vi "Update_TL_Init_Values.vi"() -> ()   [LabVIEW 2012]
uses:
  <vilib>/Utility/config.llb/Read Key (Double).vi
  <vilib>/Utility/config.llb/Write Key (Double).vi
  <vilib>/Utility/config.llb/NI_LVConfig.lvlib
panel:
  in  "Update Button":bool
  out "TL Init Values":string[](array[string])
  out "Listed\nLog Entries":string
  out "FileSize":i64
  in  "Init File Path":path=path "C:/Users/eol-lidar/Desktop/ThorLabsLog Folder/h2o_dial_settings-2.txt"
  out "bytes/line":i64
  out "FilePosition":i64
  in  "Stop":bool
  in  "Next":bool
  in  "Previous":bool
  out "ThorLabs Log Entries":string[](array[string])
  in  "ETO(mS)":i32
  in  "TL Log Entry to Write into Init File":i32=5 min=1 max=5 step=1
  out "Total\nLog Entries":dbl
  out "Error Out":errorcluster
  in  "Error In":errorcluster
  in  "TL Log File":path=path "C:/Users/eol-lidar/Desktop/ThorLabsLog Folder/TL.log"
  # "Update ThorLab Init Values"
  # "1"
  # "2"
  # "3"
  # "4"
  # "5"
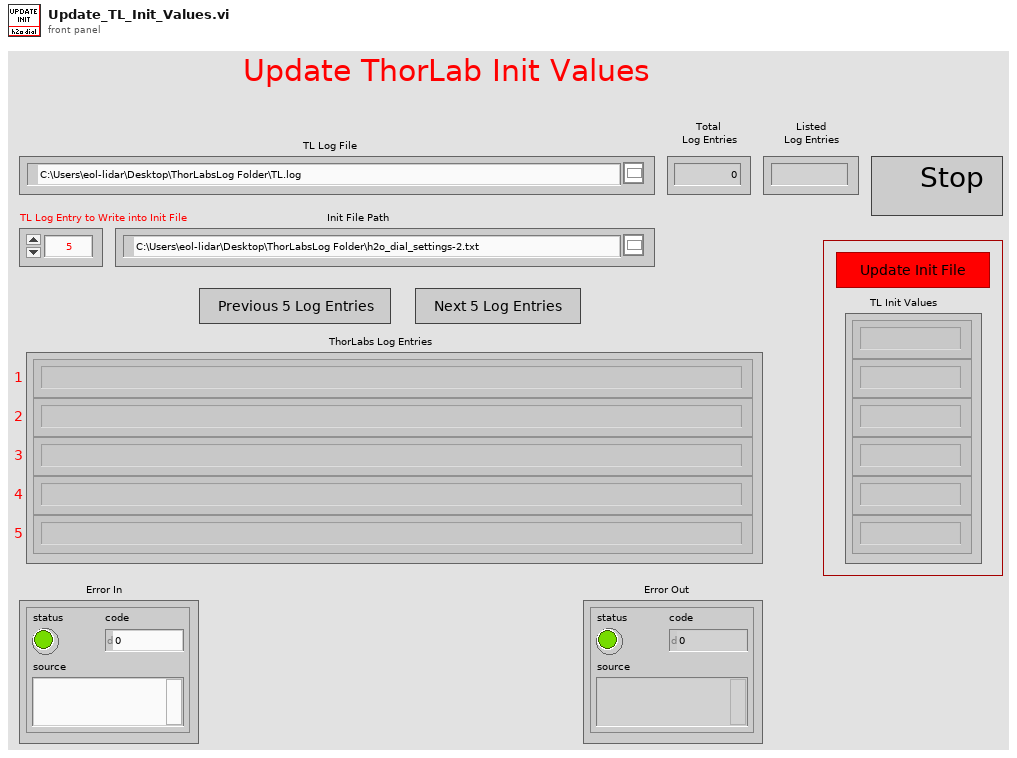
[diagram p1: front panel]
types:
  T1 = typedef "NI_LVConfig.lvlib/Config Data RefNum.ctl" = refnum<k1>
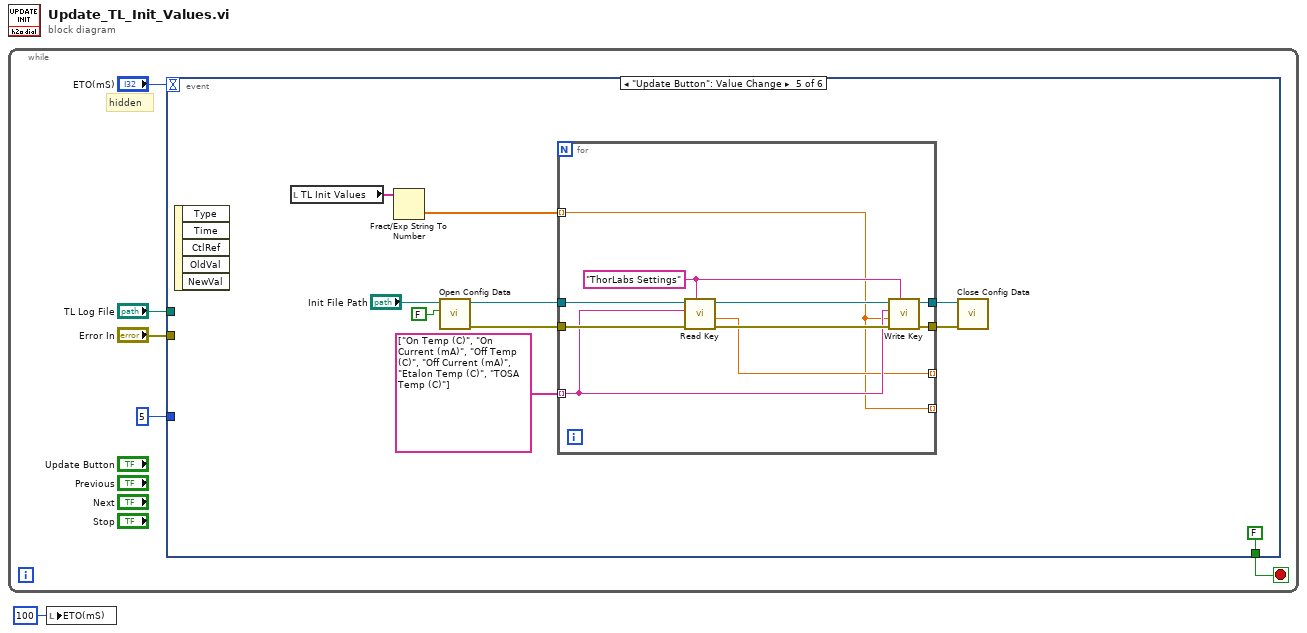
[diagram p0: block diagram]
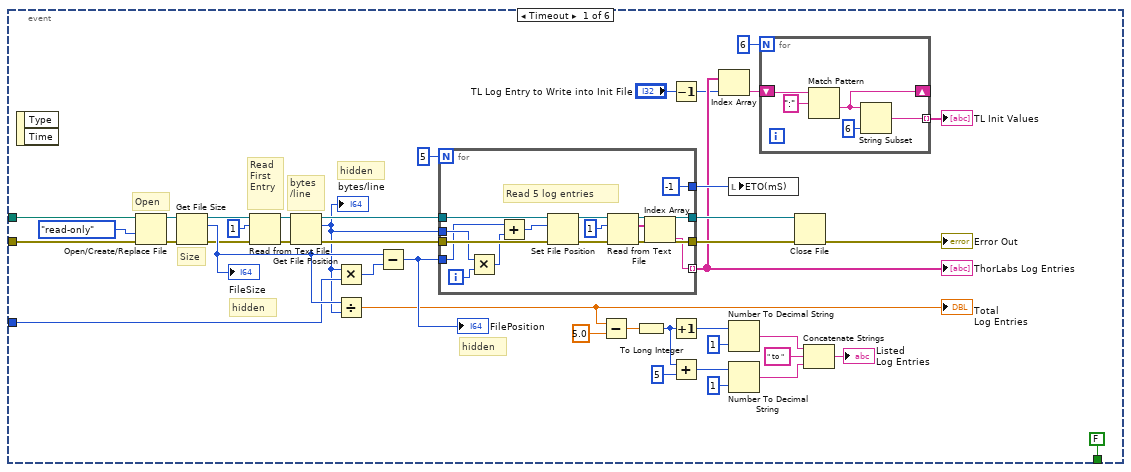
[diagram p2: hidden frame]
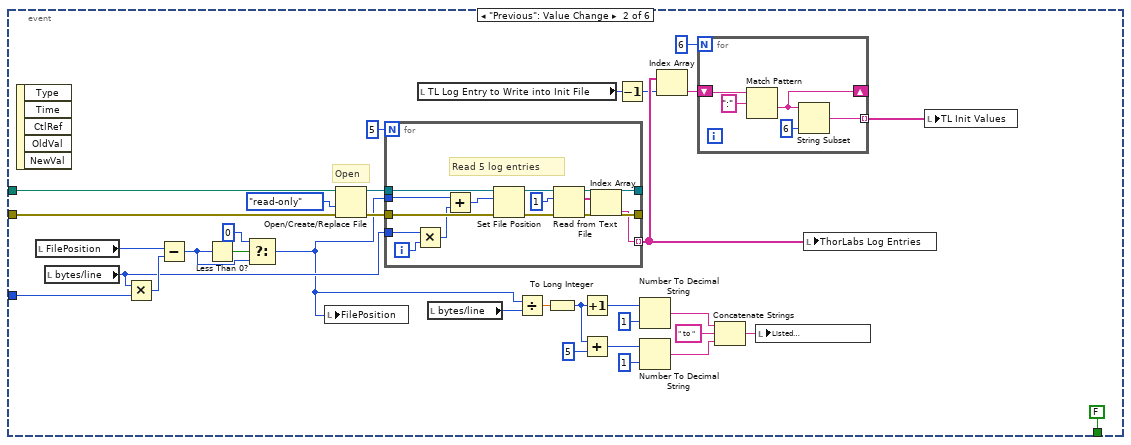
[diagram p3: hidden frame]
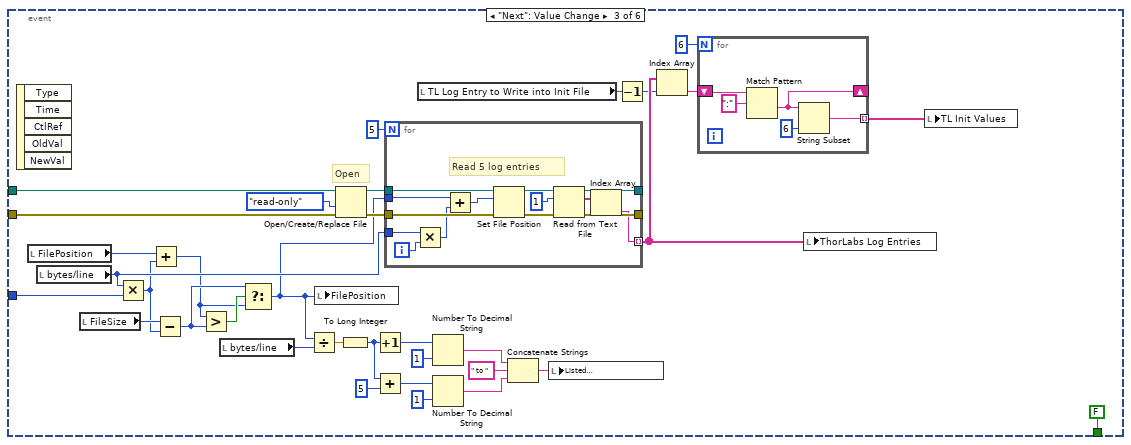
[diagram p4: hidden frame]
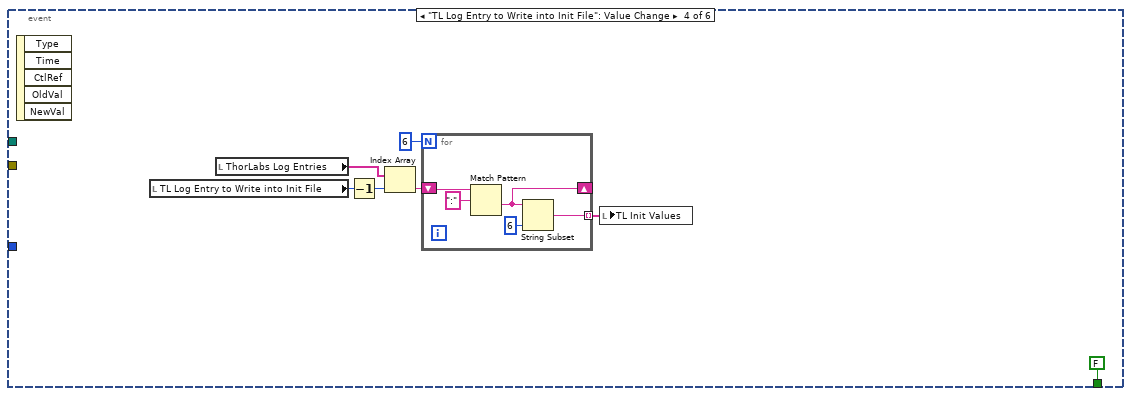
[diagram p5: hidden frame]
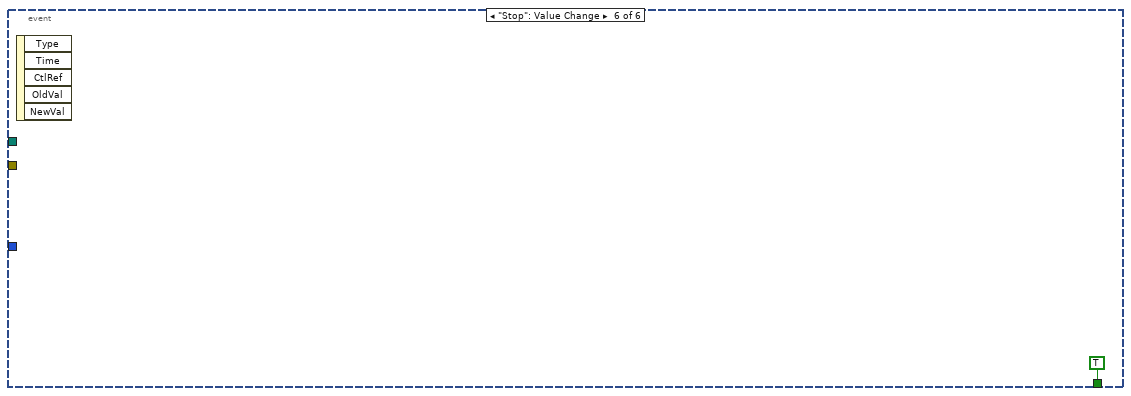
[diagram p6: hidden frame]
diagram:
  n1 = while {
    stop <- w2 stop-if-true
    # "hidden"
    n2 = event shown="[4] \"Update Button\": Value Change" {
      selector: _ -> [_ _ _ _ _ _]
      dyn-events: _ -> [_ _ _ _ _ _]
      timeout: "ETO(mS)" -> [_ _ _ _ _ _]
      tunnel: "TL Log File" -> [w32 w95 w149 _ _ _]
      tunnel: "Error In" -> [w31 w97 w151 _ _ _]
      tunnel: 5 -> [w29 w100 w153 _ _ _]
      tunnel: [FALSE FALSE FALSE FALSE FALSE TRUE] -> w2
      event Timeout {
        # "hidden"
        # "hidden"
        # "hidden"
        # "bytes\n/line"
        # "Read\nFirst\nEntry"
        # "Size"
        # "Open"
        n3 = event-data() -> ()  [unwired: 1 in, 2 out]
        n4 = Open/Create/Replace File(file path (use dialog)=w32, error in=w31, access (0:read/write)=enum16{"read/write", "read-only", "write-only"}."read-only") -> (refnum out=w34:refnum<file>, error out=w35:errorcluster)  [unwired: 3 in, 1 out]
        n5 = Get File Size(file=w34, error in=w35) -> (refnum out=w36:refnum<file>, size (in bytes)=w47:i64, 0:w37:errorcluster)
        "FileSize" <- w47
        n6 = Read from Text File(file (use dialog)=w36, count=1, error in=w37) -> (refnum out=w39:refnum<file>, error out=w38:errorcluster)  [unwired: 1 in, 2 out]
        n7 = Get File Position(4:w38, 7:w39) -> (0:w43:errorcluster, 2:w26:i64, 3:w42:refnum<file>)
        "bytes/line" <- w26
        n8 = Multiply(x=w26, y=w29) -> (x*y=w48:i64)
        n9 = Divide(x=w47, y=w26) -> (x/y=w19:dbl)
        "Total\nLog Entries" <- w19
        n10 = Subtract(x=w47, y=w48) -> (x-y=w44:i64)
        "FilePosition" <- w44
        n11 = for {
          N: 5 -> [_]
          tunnel: [w68] -> w46
          tunnel: [w67] -> w45
          tunnel: w44 -> [w56]
          tunnel: w43 -> [w65]
          tunnel: w42 -> [w64]
          tunnel: [w59] -> w25 mode=indexing
          tunnel: [-1] -> w27
          tunnel: w26 -> [w57]
          i -> [w61]
          # "Read 5 log entries"
          n12 = Multiply(x=w57, y=w61) -> (x*y=w55:i64)
          n13 = Add(x=w56, y=w55) -> (x+y=w54:i64)
          n14 = Set File Position(offset (in bytes) (0)=w54, refnum=w64, error in=w65) -> (refnum out=w63:refnum<file>, error out=w62:errorcluster)  [unwired: 1 in]
          n15 = Read from Text File(file (use dialog)=w63, count=1, error in=w62) -> (refnum out=w68:refnum<file>, text=w60:string[], error out=w67:errorcluster)  [unwired: 1 in, 1 out]
          n16 = Index Array(array=w60) -> (element=w59:string)  [unwired: 1 in]
        }
        "ThorLabs Log Entries" <- w25
        n17 = Subtract(x=w19, y=5.0) -> (x-y=w17:dbl)
        n18 = To Long Integer(number=w17) -> (32bit integer=w16:i32)
        n19 = Decrement(x="TL Log Entry to Write into Init File") -> (x-1=w20:i32)
        n20 = Increment(x=w16) -> (x+1=w12:i32)
        n21 = Add(x=w16, y=5) -> (x+y=w11:i32)
        n22 = Index Array(array=w25, index=w20) -> (element=w24:string)
        n23 = local write "ETO(mS)"(w27) -> ()
        n24 = Number To Decimal String(number=w12, width (-)=i16 1) -> (decimal integer string=w10:string)
        n25 = Number To Decimal String(number=w11, width (-)=i16 1) -> (decimal integer string=w8:string)
        n26 = for {
          N: 6 -> [_]
          tunnel: [w51] -> w23 mode=indexing
          shift-right: [w50] -> _
          shift-left: w24 -> [w49]
          n27 = Match Pattern(string=w49, regular expression=":") -> (after substring=w50:string)  [unwired: 1 in, 3 out]
          n28 = String Subset(string=w50, length (rest)=6 ("length (rest)")) -> (substring=w51:string)  [unwired: 1 in]
        }
        "TL Init Values" <- w23
        n29 = Close File(refnum=w46, error in=w45) -> (error out=→"Error Out":errorcluster)  [unwired: 1 out]
        n30 = Concatenate Strings(w10, " to " ("string"), w8) -> (→"Listed\nLog Entries":string)
      }
      event "Previous": Value Change {
        # "Open"
        n31 = event-data() -> ()  [unwired: 1 in, 5 out]
        n32 = local read "FilePosition"() -> (w101:i64)
        n33 = local read "bytes/line"() -> (w93:i64)
        n34 = Multiply(x=w93, y=w100) -> (x*y=w99:i64)
        n35 = Subtract(x=w101, y=w99) -> (x-y=w83:i64)
        n36 = Less Than 0?(x=w83) -> (x < 0?=w84:bool)
        n37 = Select(t=0, s=w84, f=w83) -> (s? t:f=w81:i64)
        n38 = local write "FilePosition"(w81) -> ()
        n39 = Open/Create/Replace File(file path (use dialog)=w95, error in=w97, access (0:read/write)=enum16{"read/write", "read-only", "write-only"}."read-only") -> (refnum out=w94:refnum<file>, error out=w96:errorcluster)  [unwired: 3 in, 1 out]
        n40 = for {
          N: 5 -> [_]
          tunnel: [w120] -> _
          tunnel: [w119] -> _
          tunnel: w81 -> [w109]
          tunnel: w96 -> [w117]
          tunnel: w94 -> [w116]
          tunnel: [w111] -> w87 mode=indexing
          tunnel: w93 -> [w110]
          i -> [w113]
          # "Read 5 log entries"
          n41 = Multiply(x=w110, y=w113) -> (x*y=w108:i64)
          n42 = Add(x=w109, y=w108) -> (x+y=w107:i64)
          n43 = Set File Position(offset (in bytes) (0)=w107, refnum=w116, error in=w117) -> (refnum out=w115:refnum<file>, error out=w114:errorcluster)  [unwired: 1 in]
          n44 = Read from Text File(file (use dialog)=w115, count=1, error in=w114) -> (refnum out=w120:refnum<file>, text=w112:string[], error out=w119:errorcluster)  [unwired: 1 in, 1 out]
          n45 = Index Array(array=w112) -> (element=w111:string)  [unwired: 1 in]
        }
        n46 = local read "TL Log Entry to Write into Init File"() -> (w89:i32)
        n47 = local read "bytes/line"() -> (w80:i64)
        n48 = Divide(x=w81, y=w80) -> (x/y=w69:dbl)
        n49 = To Long Integer(number=w69) -> (32bit integer=w79:i32)
        n50 = Increment(x=w79) -> (x+1=w75:i32)
        n51 = Add(x=w79, y=5) -> (x+y=w74:i32)
        n52 = Decrement(x=w89) -> (x-1=w85:i32)
        n53 = Number To Decimal String(number=w75, width (-)=i16 1) -> (decimal integer string=w73:string)
        n54 = Number To Decimal String(number=w74, width (-)=i16 1) -> (decimal integer string=w71:string)
        n55 = Index Array(array=w87, index=w85) -> (element=w91:string)
        n56 = for {
          N: 6 -> [_]
          tunnel: [w104] -> w86 mode=indexing
          shift-right: [w103] -> _
          shift-left: w91 -> [w102]
          n57 = Match Pattern(string=w102, regular expression=":") -> (after substring=w103:string)  [unwired: 1 in, 3 out]
          n58 = String Subset(string=w103, length (rest)=6 ("length (rest)")) -> (substring=w104:string)  [unwired: 1 in]
        }
        n59 = Concatenate Strings(w73, " to " ("string"), w71) -> (w70:string)
        n60 = local write "Listed\nLog Entries"(w70) -> ()
        n61 = local write "ThorLabs Log Entries"(w87) -> ()
        n62 = local write "TL Init Values"(w86) -> ()
      }
      event "Next": Value Change {
        # "Open"
        n63 = event-data() -> ()  [unwired: 1 in, 5 out]
        n64 = local read "FilePosition"() -> (w154:i64)
        n65 = local read "bytes/line"() -> (w147:i64)
        n66 = local read "FileSize"() -> (w137:i64)
        n67 = Multiply(x=w147, y=w153) -> (x*y=w136:i64)
        n68 = Add(x=w154, y=w136) -> (x+y=w134:i64)
        n69 = Subtract(x=w137, y=w136) -> (x-y=w135:i64)
        n70 = Greater?(x=w134, y=w135) -> (0:w138:bool)
        n71 = local read "bytes/line"() -> (w133:i64)
        n72 = Select(t=w135, s=w138, f=w134) -> (s? t:f=w132:i64)
        n73 = Divide(x=w132, y=w133) -> (x/y=w121:dbl)
        n74 = local write "FilePosition"(w132) -> ()
        n75 = Open/Create/Replace File(file path (use dialog)=w149, error in=w151, access (0:read/write)=enum16{"read/write", "read-only", "write-only"}."read-only") -> (refnum out=w148:refnum<file>, error out=w150:errorcluster)  [unwired: 3 in, 1 out]
        n76 = To Long Integer(number=w121) -> (32bit integer=w123:i32)
        n77 = Increment(x=w123) -> (x+1=w122:i32)
        n78 = Add(x=w123, y=5) -> (x+y=w128:i32)
        n79 = for {
          N: 5 -> [_]
          tunnel: [w173] -> _
          tunnel: [w172] -> _
          tunnel: w132 -> [w162]
          tunnel: w150 -> [w170]
          tunnel: w148 -> [w169]
          tunnel: [w164] -> w141 mode=indexing
          tunnel: w147 -> [w163]
          i -> [w166]
          # "Read 5 log entries"
          n80 = Multiply(x=w163, y=w166) -> (x*y=w161:i64)
          n81 = Add(x=w162, y=w161) -> (x+y=w160:i64)
          n82 = Set File Position(offset (in bytes) (0)=w160, refnum=w169, error in=w170) -> (refnum out=w168:refnum<file>, error out=w167:errorcluster)  [unwired: 1 in]
          n83 = Read from Text File(file (use dialog)=w168, count=1, error in=w167) -> (refnum out=w173:refnum<file>, text=w165:string[], error out=w172:errorcluster)  [unwired: 1 in, 1 out]
          n84 = Index Array(array=w165) -> (element=w164:string)  [unwired: 1 in]
        }
        n85 = local read "TL Log Entry to Write into Init File"() -> (w143:i32)
        n86 = Number To Decimal String(number=w122, width (-)=i16 1) -> (decimal integer string=w127:string)
        n87 = Number To Decimal String(number=w128, width (-)=i16 1) -> (decimal integer string=w125:string)
        n88 = Concatenate Strings(w127, " to " ("string"), w125) -> (w124:string)
        n89 = local write "Listed\nLog Entries"(w124) -> ()
        n90 = Decrement(x=w143) -> (x-1=w139:i32)
        n91 = Index Array(array=w141, index=w139) -> (element=w145:string)
        n92 = for {
          N: 6 -> [_]
          tunnel: [w157] -> w140 mode=indexing
          shift-right: [w156] -> _
          shift-left: w145 -> [w155]
          n93 = Match Pattern(string=w155, regular expression=":") -> (after substring=w156:string)  [unwired: 1 in, 3 out]
          n94 = String Subset(string=w156, length (rest)=6 ("length (rest)")) -> (substring=w157:string)  [unwired: 1 in]
        }
        n95 = local write "ThorLabs Log Entries"(w141) -> ()
        n96 = local write "TL Init Values"(w140) -> ()
      }
      event "TL Log Entry to Write into Init File": Value Change {
        n97 = event-data() -> ()  [unwired: 1 in, 5 out]
        n98 = local read "TL Log Entry to Write into Init File"() -> (w180:i32)
        n99 = local read "ThorLabs Log Entries"() -> (w179:string[])
        n100 = Decrement(x=w180) -> (x-1=w175:i32)
        n101 = Index Array(array=w179, index=w175) -> (element=w177:string)
        n102 = for {
          N: 6 -> [_]
          tunnel: [w183] -> w176 mode=indexing
          shift-right: [w182] -> _
          shift-left: w177 -> [w181]
          n103 = Match Pattern(string=w181, regular expression=":") -> (after substring=w182:string)  [unwired: 1 in, 3 out]
          n104 = String Subset(string=w182, length (rest)=6 ("length (rest)")) -> (substring=w183:string)  [unwired: 1 in]
        }
        n105 = local write "TL Init Values"(w176) -> ()
      }
      event "Update Button": Value Change {
        n106 = event-data() -> ()  [unwired: 1 in, 5 out]
        n107 = local read "TL Init Values"() -> (w189:string[])
        n108 = Fract/Exp String To Number(string=w189) -> (number=w188:dbl[])  [unwired: 3 in, 1 out]
        n109 = call <vilib>:"Open Config Data.vi"("create file if necessary (T)"=FALSE, "configuration file path"="Init File Path") -> ("error out"=w192:errorcluster, "refnum"=w194:T1)  [unwired: 7 in, 1 out]
        n110 = for {
          tunnel: w194 -> [w205]
          tunnel: [w202] -> w193
          tunnel: w192 -> [w204]
          tunnel: [w200] -> w191
          tunnel: string[] ["On Temp (C)", "On Current (mA)", "Off Temp (C)", "Off Current (mA)", "Etalon Temp (C)", "TOSA Temp (C)"] ("Array 3") -> [w199] mode=indexing
          tunnel: [w198] -> _ mode=indexing
          tunnel: [w196] -> _ mode=indexing
          tunnel: w188 -> [w196] mode=indexing
          w197 = "ThorLabs Settings"
          n111 = call-poly <vilib>:"Read Key.vi"("section"=w197, "error in (no error)"=w204, "key"=w199, "refnum"=w205) -> ("error out"=w201:errorcluster, "value"=w198:dbl, "refnum out"=w203:T1)  [unwired: 4 in, 1 out]
          n112 = call-poly <vilib>:"Write Key.vi"("section"=w197, "error in (no error)"=w201, "value"=w196, "key"=w199, "refnum"=w203) -> ("error out"=w200:errorcluster, "refnum out"=w202:T1)  [unwired: 4 in, 1 out]
        }
        n113 = call <vilib>:"Close Config Data.vi"("error in (no error)"=w191, "refnum"=w193) -> ()  [unwired: 8 in, 2 out]
      }
      event "Stop": Value Change {
        n114 = event-data() -> ()  [unwired: 1 in, 5 out]
      }
    }
  }
  n115 = local write "ETO(mS)"(100 ("ETO(mS)")) -> ()
